vi "go home.vi"(8 "error in (no error)":errorcluster, 9 "HOME":bool, 10 "DELAY (ms) in":u32, 11 "VISA Refnum in":refnum<visa-resource-name>) -> (1 "error out":errorcluster, 2 "DELAY (ms) out":u32, 3 "Dup. VISA handle":refnum<visa-resource-name>)   [LabVIEW 2014]
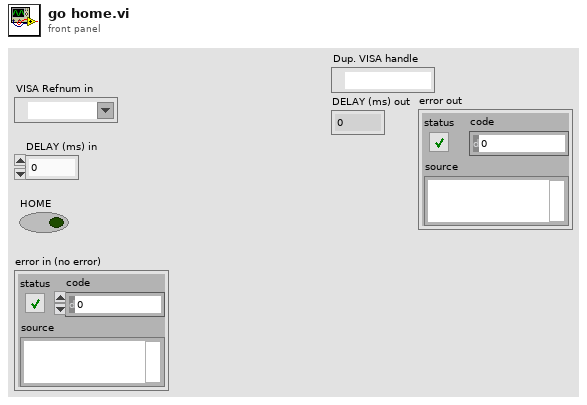
[diagram p1: front panel]
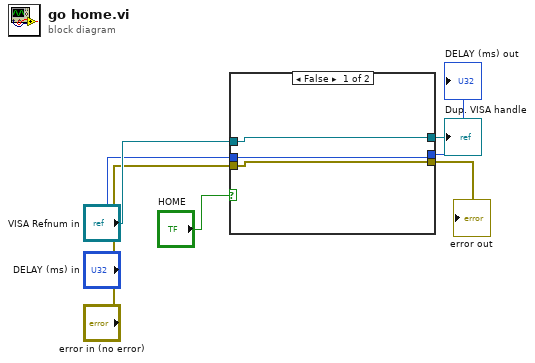
[diagram p0: block diagram]
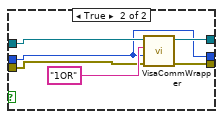
[diagram p2: hidden frame]
diagram:
  n1 = case shown="False" "HOME" {
    tunnel: "DELAY (ms) in" -> [w9 w11]
    tunnel: "error in (no error)" -> [w8 w14]
    tunnel: "VISA Refnum in" -> [w10 w16]
    tunnel: [w8 w13] -> w1
    tunnel: [w10 w12] -> w3
    tunnel: [w9 w11] -> w2
    frame False {
    }
    frame True {
      n2 = call <userlib>:"VisaCommWrapper.vi"("error in (no error)"=w14, "Delay (ms)"=w11, "Command"="1OR", "VISA handle"=w16) -> ("error out"=w13:errorcluster, "Dup. VISA handle"=w12:refnum<visa-resource-name>)  [unwired: 1 in, 3 out]
    }
  }
  "Dup. VISA handle" <- w3
  "DELAY (ms) out" <- w2
  "error out" <- w1
